vi "SetCP.vi"(3 "error in (no error)":errorcluster, 4 "CP(=RTS) state":i16 min=0 max=1 step=1, 5 "VISA resource":refnum<visa-resource-name>="COM1") -> (0 "error out":errorcluster, 2 "dup VISA resource":refnum<visa-resource-name>="COM1")   [LabVIEW 2021]
doc: "Controls state of clock signal\nto AVS-47B"
panel:
  # "SetCP.vi"
  # "This VI controls the state (1 or 0)  of the CP (Clock Pulse) Picobus output  line (RTS handshake of the COM port)."
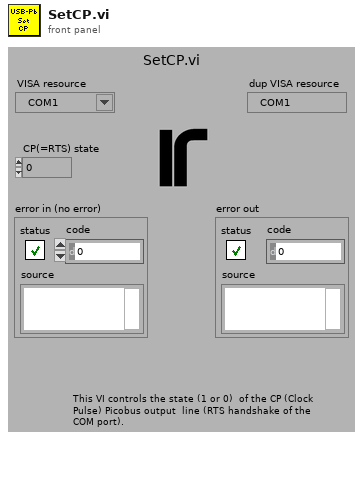
[diagram p1: front panel]
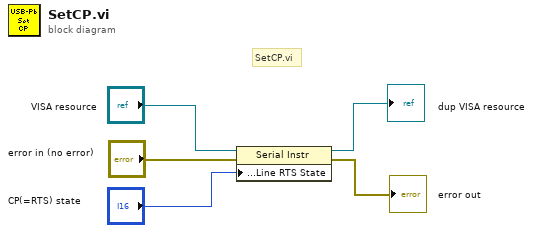
[diagram p0: block diagram]
diagram:
  # "SetCP.vi"
  n1 = property class="Serial Instr"(reference="VISA resource", error in="error in (no error)", "Serial Settings:Modem Line Settings:Line RTS State"="CP(=RTS) state") -> (reference out=→"dup VISA resource":refnum<visa-resource-name>, error out=→"error out":errorcluster)
